vi "Native labview GET.vi"() -> ()   [LabVIEW 2017]
uses:
  Bridge Configuration.ctl
  <vilib>/httpClient/LabVIEWHTTPClient.lvlib
panel:
  out "error out":errorcluster
  out "Parsed bridge configuration":T1
  in  "Base URL":string="http://localhost:3000/bridge"
  out "Returned body":string
  out "Returned headers":string
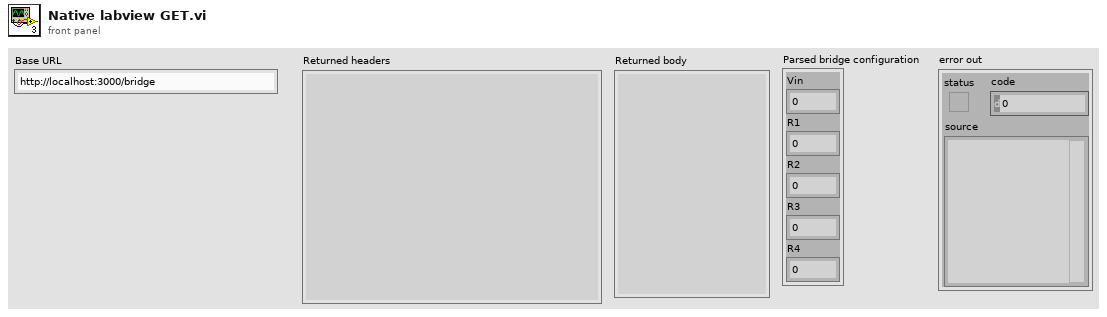
[diagram p1: front panel]
types:
  T1 = typedef "Bridge Configuration.ctl" = cluster{"Vin":dbl, "R1":dbl, "R2":dbl, "R3":dbl, "R4":dbl}
  T2 = typedef "LabVIEWHTTPClient.lvlib/ClientHandle.ctl" = refnum<k1>
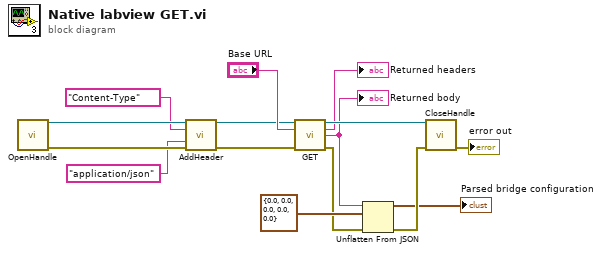
[diagram p0: block diagram]
diagram:
  n1 = call <vilib>:"OpenHandle.vi"() -> ("client handle out"=w12:T2, "error out"=w11:errorcluster)  [unwired: 14 in]
  n2 = call <vilib>:"AddHeader.vi"("client handle"=w12, "header"="Content-Type", "value"="application/json", "error in (no error)"=w11) -> ("client handle out"=w8:T2, "error out"=w7:errorcluster)  [unwired: 10 in]
  n3 = call <vilib>:"GET.vi"("client handle"=w8, "url"="Base URL", "error in (no error)"=w7) -> ("client handle out"=w15:T2, "headers"=→"Returned headers":string, "body"=w5:string, "error out"=w4:errorcluster)  [unwired: 9 in]
  "Returned body" <- w5
  n4 = Unflatten From JSON(JSON string=w5, type and defaults=T1 {"Vin"=0.0, "R1"=0.0, "R2"=0.0, "R3"=0.0, "R4"=0.0} ("Bridge Configuration"), error in (no error)=w4) -> (value=→"Parsed bridge configuration":T1, error out=w3:errorcluster)  [unwired: 4 in]
  n5 = call <vilib>:"CloseHandle.vi"("client handle"=w15, "error in (no error)"=w3) -> ("error out"=→"error out":errorcluster)  [unwired: 13 in]
